vi "Sub Initialize.vi"(8 "error in (no error)":errorcluster, 11 "Instrument Recorder in":refnum<class "Micron Optics Recorder.lvclass">) -> (0 "error out":errorcluster, 2 "Initialize Result":refnum<class "Acquired Result.lvclass">, 3 "Instrument Recorder out":refnum<class "Micron Optics Recorder.lvclass">)   [LabVIEW 2016, in "Micron Optics Recorder.lvclass"]
uses:
  Micron Optics Recorder.lvclass
  C:/github/Measure_core/Template Module/Template Module.lvclass
  Measure_core/Results/Acquired Result/Acquired Result.lvclass
  NHMFL_Core/Libraries/Instruments/Micron Optics/Micron optics configuration.ctl
  Measure_core/Template Module/Template Module.lvclass/Template Module.ctl
  NHMFL_Core/Libraries/Instruments/Micron Optics/Micron Optics Driver/Micron Optics Driver.lvclass/Micron Optics Driver.ctl
  Measure_core/Template Module/Read Configuration.vi
  NHMFL_Core/Libraries/Instruments/Micron Optics/Micron Optics Driver/Write Configuration.vi
  Read Micron Optics Driver.vi
  Write Micron Optics Driver.vi
  NHMFL_Core/Libraries/Instruments/Micron Optics/Micron Optics Driver/Micron Optics Driver.lvclass
  Measure_core/Instrument Actor/Instrument Actor.lvclass
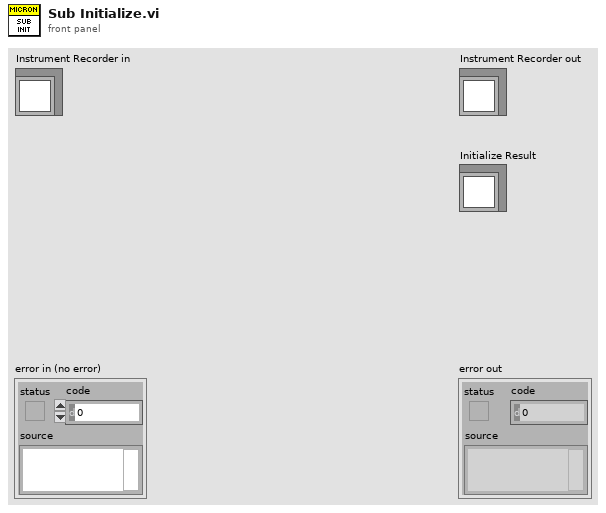
[diagram p1: front panel]
types:
  T1 = typedef "Micron optics configuration.ctl" = cluster{"Reference channel":i32, "Detection Setting ID":u8, "Address":string}
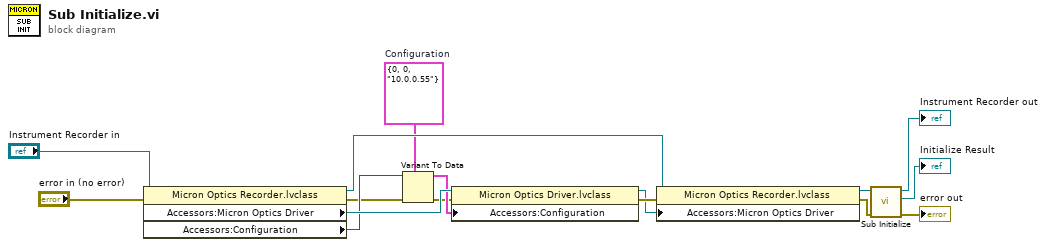
[diagram p0: block diagram]
diagram:
  w8 = T1 {"Reference channel"=0, "Detection Setting ID"=0, "Address"="10.0.0.55"}  # Configuration
  n1 = property class="Micron Optics Recorder.lvclass"(reference="Instrument Recorder in", error in="error in (no error)") -> (reference out=w11:refnum<class "Micron Optics Recorder.lvclass">, error out=w5:errorcluster, "Accessors:Micron Optics Driver"=w10:refnum<class "Micron Optics Driver.lvclass">, "Accessors:Configuration"=w9:variant)
  n2 = Variant To Data(error in=w5, type=w8, Variant=w9) -> (data=w7:T1, error out=w6:errorcluster)
  n3 = property class="Micron Optics Driver.lvclass"(reference=w10, error in=w6, "Accessors:Configuration"=w7) -> (reference out=w2:refnum<class "Micron Optics Driver.lvclass">, error out=w3:errorcluster)
  n4 = property class="Micron Optics Recorder.lvclass"(reference=w11, error in=w3, "Accessors:Micron Optics Driver"=w2) -> (reference out=w4:refnum<class "Micron Optics Recorder.lvclass">, error out=w1:errorcluster)
  n5 = call-parent "Sub Initialize.vi"("error in (no error)"=w1, "Instrument Recorder in"=w4) -> ("error out"=→"error out":errorcluster, "Initialize Result"=→"Initialize Result":refnum<class "Acquired Result.lvclass">, "Instrument Recorder out"=→"Instrument Recorder out":refnum<class "Micron Optics Recorder.lvclass">)  [unwired: 7 in]
